vi "Operaciones comparativas.vi"() -> ()   [LabVIEW 2022 SP3]
panel:
  out "Indicador 2":string
  out "Indicador 1":string
  out "Alarma 2":bool
  out "Alarma 1":bool
  in  "Umbral para T1K 2":u8(slide) scale=0.0..100.0
  in  "Gauge 2":dbl(knob) scale=0.0..100.0
  out "Termocupla 2 tipo k 2":dbl(slide) scale=0.0..100.0
  in  "Umbral para T1K":u8(slide) scale=0.0..100.0
  in  "Gauge":dbl(knob) scale=0.0..100.0
  out "Termocupla 1 tipo k":dbl(slide) scale=0.0..100.0
  # "Se tiene 2 termocuplas tipo k en cual se estara simuladno de manera manual por medio de dos controles\ndbl c/u\n\nSe desea:\nA) Para cada termocupla activar una alarma cuando este pase un umbral establesido\nB) Si la temperatura es mayor e igual al umbral establesido entonces, mostraremos en un indicador string \nel siguiente mensaje, \"que la temperatura esta fuera de rango\" y asu vez activar una alarma, caso contrario \nsi es menor al umbral mostrar en el mismo indicador string(\"estable\")"
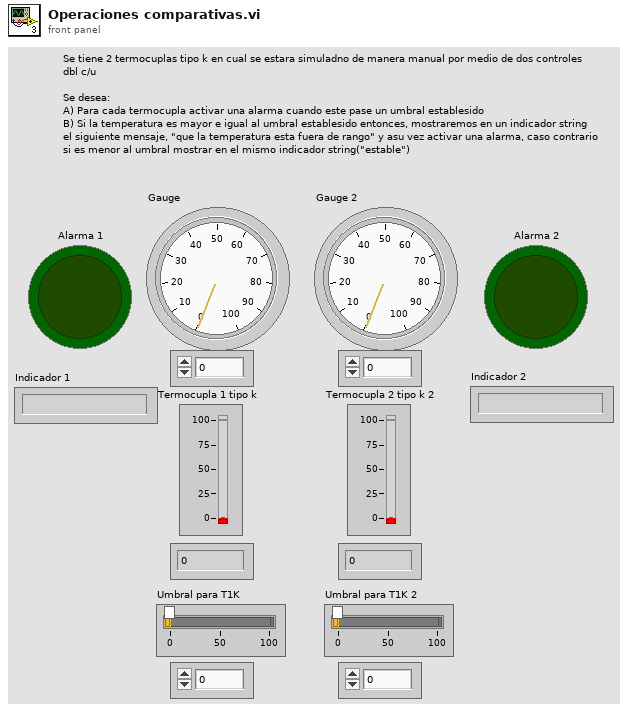
[diagram p1: front panel]
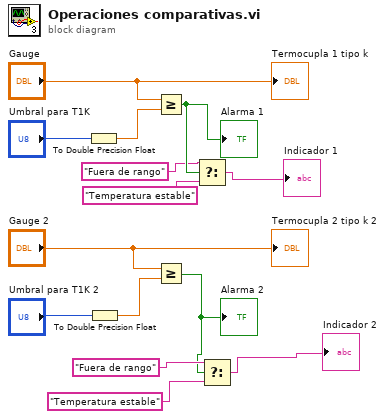
[diagram p0: block diagram]
diagram:
  n1 = To Double Precision Float(number="Umbral para T1K") -> (double precision float=w10:dbl)
  n2 = To Double Precision Float(number="Umbral para T1K 2") -> (double precision float=w9:dbl)
  n3 = Greater Or Equal?(x="Gauge", y=w10) -> (x >= y?=w8:bool)
  "Alarma 1" <- w8
  n4 = Greater Or Equal?(x="Gauge 2", y=w9) -> (x >= y?=w2:bool)
  "Alarma 2" <- w2
  n5 = Select(t="Fuera de rango", s=w8, f="Temperatura estable") -> (s? t:f=→"Indicador 1":string)
  n6 = Select(t="Fuera de rango", s=w2, f="Temperatura estable") -> (s? t:f=→"Indicador 2":string)
  "Termocupla 1 tipo k" <- "Gauge"
  "Termocupla 2 tipo k 2" <- "Gauge 2"
